vi "CreateErrorLog.vi"() -> (3 "path":path)   [LabVIEW 2012]
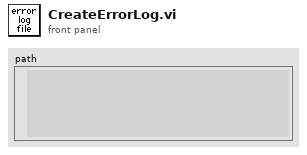
[diagram p1: front panel]
types:
  T1 = enum16{"open", "replace", "create", "open or create", "replace or create", "replace or create with confirmation"}
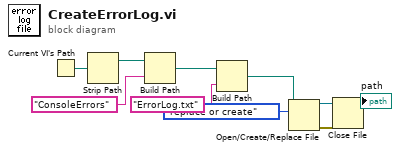
[diagram p0: block diagram]
diagram:
  n1 = Current VI's Path() -> (path=w5:path)
  n2 = Strip Path(path=w5) -> (stripped path=w6:path)  [unwired: 1 out]
  n3 = Build Path(base path=w6, name or relative path="ConsoleErrors") -> (appended path=w8:path)
  n4 = Build Path(base path=w8, name or relative path="ErrorLog.txt") -> (appended path=w10:path)
  n5 = Open/Create/Replace File(file path (use dialog)=w10, operation (0:open)=T1."replace or create") -> (refnum out=w3:refnum<file>, error out=w2:errorcluster)  [unwired: 4 in, 1 out]
  n6 = Close File(refnum=w3, error in=w2) -> (path=→"path":path)  [unwired: 1 out]
